vi "......SPEECH + GAIT + FACE  two command.vi"() -> ()   [LabVIEW 2018]
uses:
  <vilib>/Analysis/baseanly.llb/Mean (DBL).vi
  <vilib>/University of Leeds/Kinesthesia Toolkit for Microsoft Kinect/_Polymorphic Configure/Event-Skeleton and Video.vi
  <vilib>/Utility/file.llb/Read Delimited Spreadsheet (DBL).vi
  <vilib>/University of Leeds/Kinesthesia Toolkit for Microsoft Kinect/_Polymorphic Read/Read-Skeleton and Video.vi
  <vilib>/University of Leeds/Kinesthesia Toolkit for Microsoft Kinect/_Polymorphic Close/Close-Skeleton and Video.vi
  <vilib>/University of Leeds/Kinesthesia Toolkit for Microsoft Kinect/_Polymorphic Configure/Event-Video.vi
  <vilib>/University of Leeds/Kinesthesia Toolkit for Microsoft Kinect/_Polymorphic Read/Read-Video.vi
  <vilib>/University of Leeds/Kinesthesia Toolkit for Microsoft Kinect/_Polymorphic Close/Close-Video.vi
  <vilib>/Utility/file.llb/Write Delimited Spreadsheet (DBL).vi
  <vilib>/Analysis/NI_AALBase.lvlib
  <vilib>/vision/NI_Vision_Development_Module.lvlib
panel:
  in  "Eye Min Score":sgl=700.0
  in  "Nose Min Score":sgl=700.0
  in  "Lip Min Score":sgl=700.0
  out "Preview":T1(plugin-control)
  in  "Show Templates":bool
  out "Face Recognized?":bool
  out "Eye Template":T1(plugin-control)
  out "Nose Template":T1(plugin-control)
  out "Lips Template":T1(plugin-control)
  out "scan gait":refnum<vi>(3d-picture)
  out "Gait recognized?":bool
  out "real time data":dbl[](array[numeric])
  out "max mean":dbl[][](array[numeric])
  out "min mean":dbl[][](array[numeric])
  out "score":dbl
  out "mean calculated":dbl[](array[numeric])
  out "measure 3D":refnum<vi>(3d-picture)
  out "measure 2D":picture
  out "real time data":dbl[](array[numeric])
  in  "Error In":errorcluster
  out "Error Out":errorcluster
  in  "Exit":bool
  out "Speech Recognition":string
  # "Gait recognition"
  # "Set up user Gait info"
  # "Face recognition"
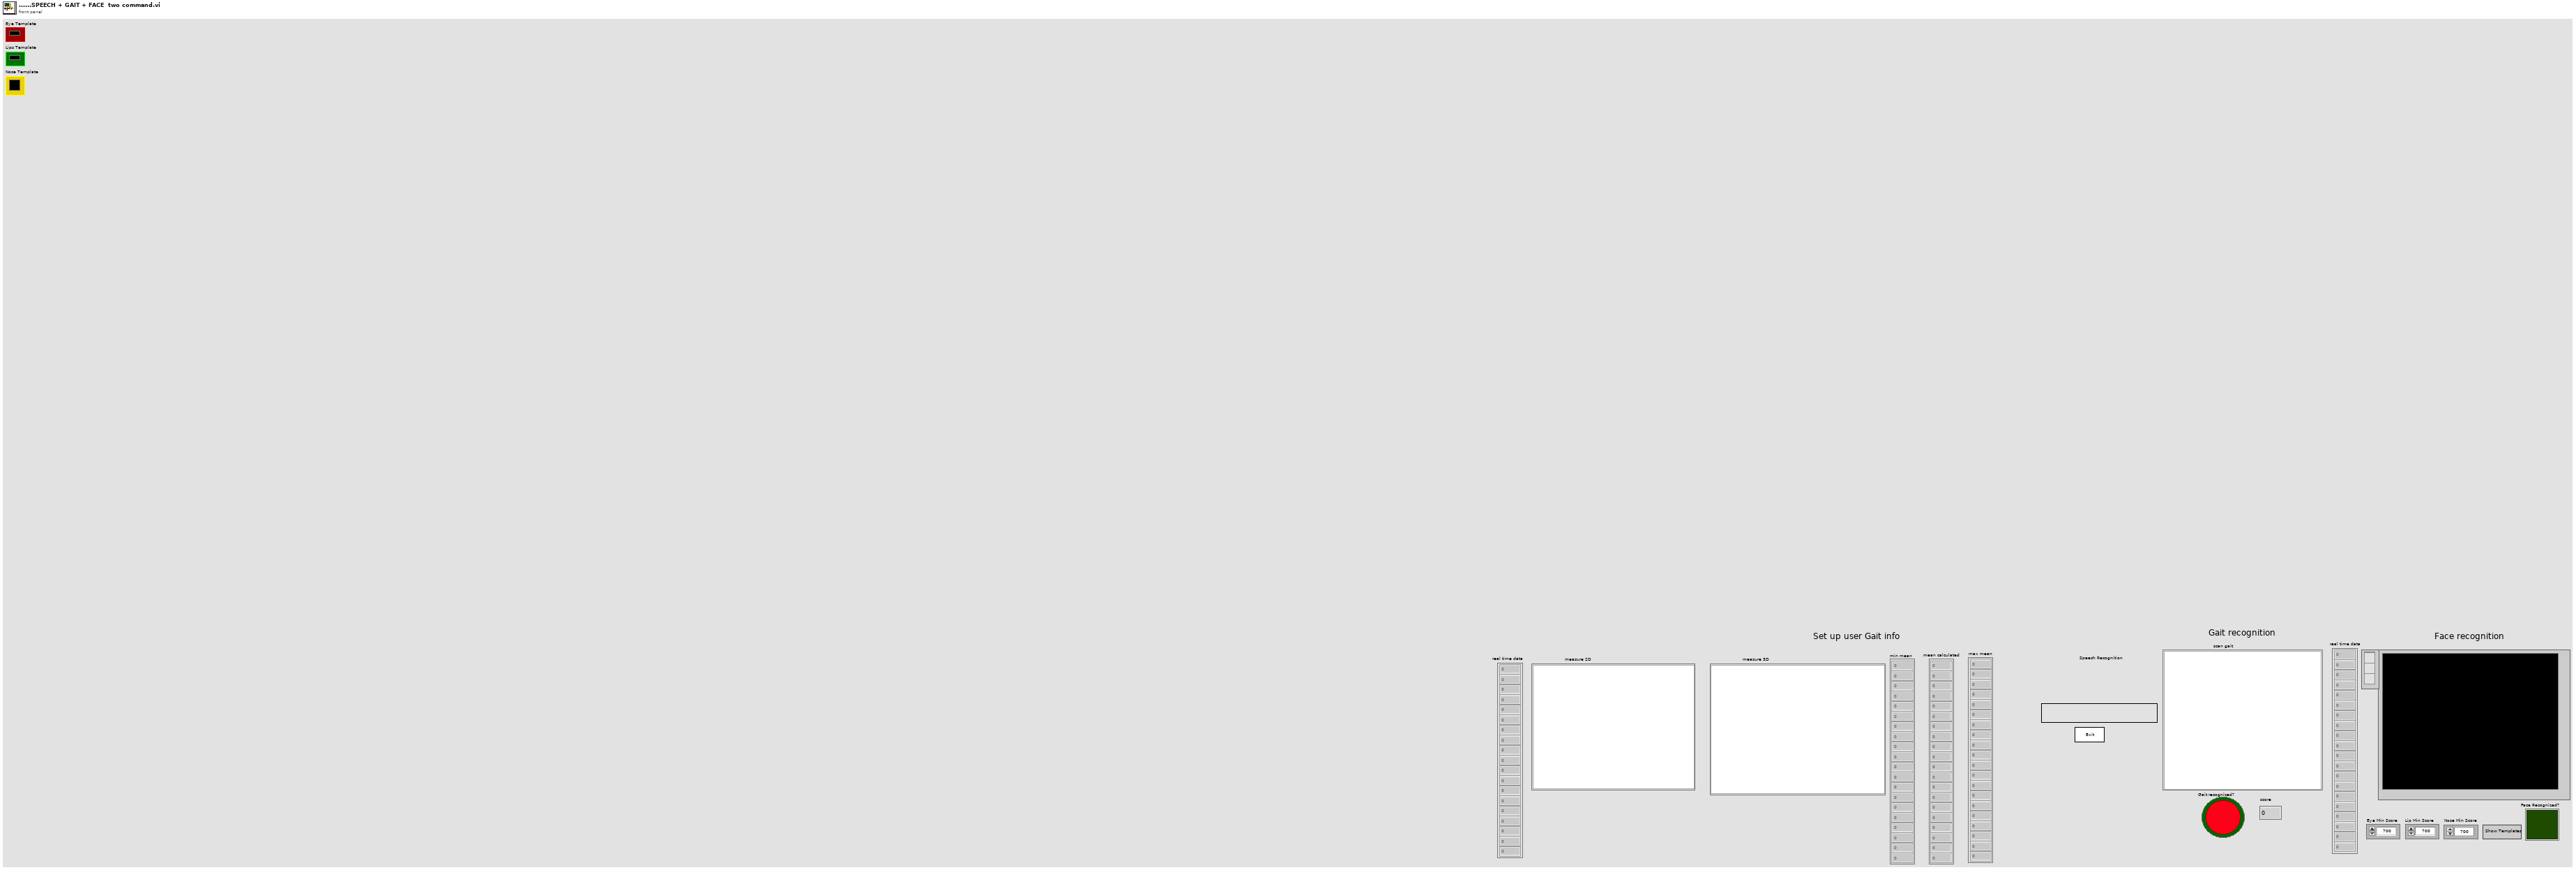
[diagram p1: front panel]
types:
  T1 = typedef "IMAQ Image.ctl" = refnum<image>
  T2 = enum16{"hip centre", "spine", "shoulder centre", "head", "shoulder left", "elbow left", "wrist left", "hand left", "shoulder right", "elbow right", "wrist right", "hand right", "hip left", "knee left", "ankle left", "foot left", "hip right", "knee right", "ankle right", "foot right"}
  T3 = cluster{cluster{"reference out":refnum<k24>, "KinectSensors":refnum<k24>}, "get_Item":refnum<k24>}
  T4 = cluster{"reference out":refnum<k24>, "KinectSensors":refnum<k24>, "SkeletonStream":refnum<k24>, "ColorStream":refnum<k24>, refnum<k24>[], "get_Item":refnum<k24>}
  T5 = cluster{"Scene":refnum<vi>, "Joints":refnum<vi>[], "Bones":refnum<vi>[]}
  T6 = cluster{"reference out":refnum<k24>, "KinectSensors":refnum<k24>, "ColorStream":refnum<k24>, "get_Item":refnum<k24>}
  T7 = typedef "Image Type" = u32
  T8 = cluster{"Position":cluster{"x":sgl, "y":sgl}, "Angle":sgl, "Scale":sgl, "Score":sgl, "Bounding Box":cluster{"x":sgl, "y":sgl}[]}[]
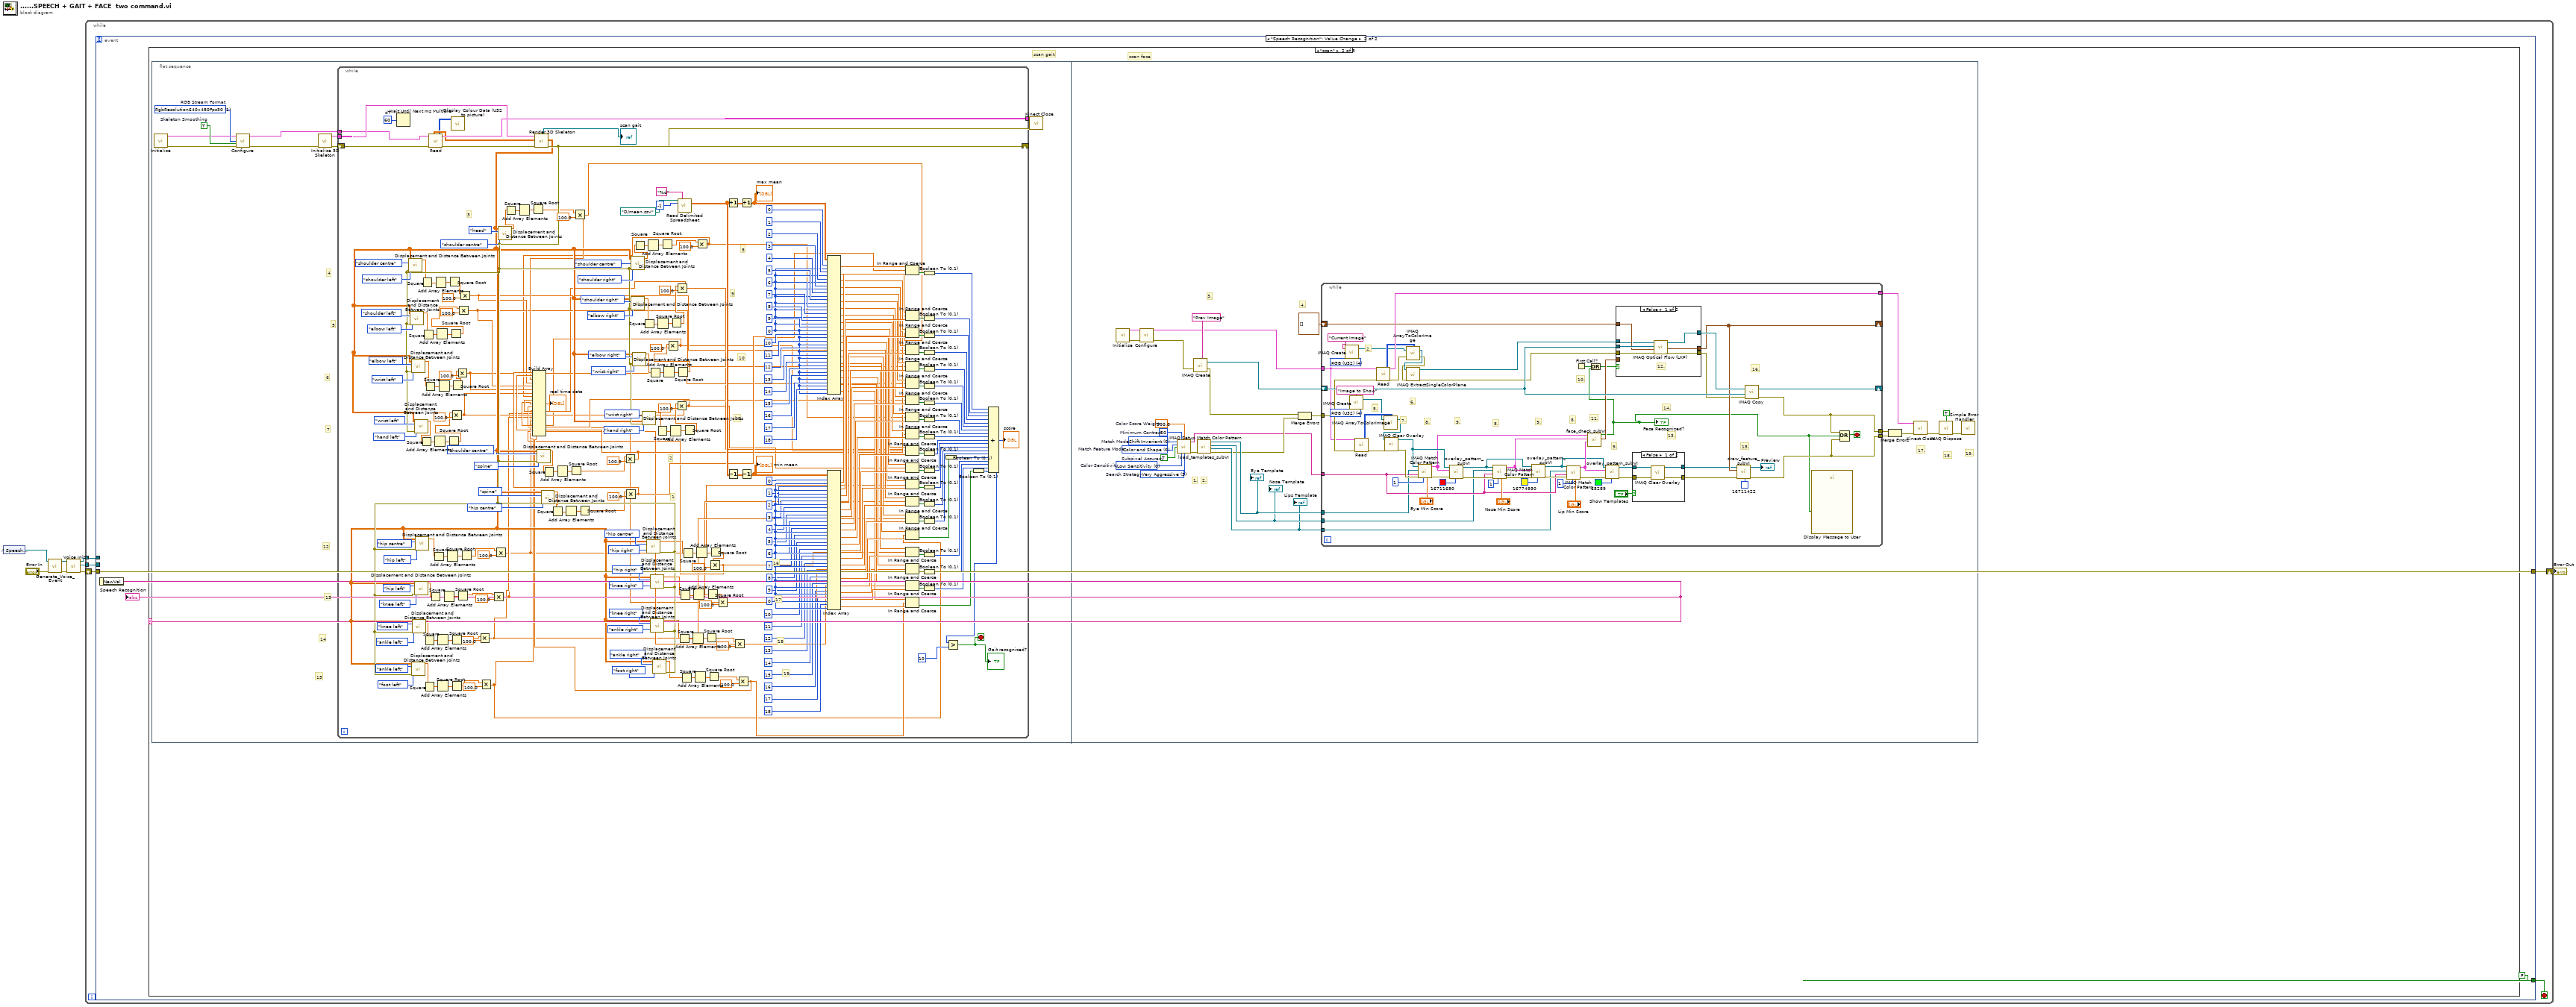
[diagram p0: block diagram]
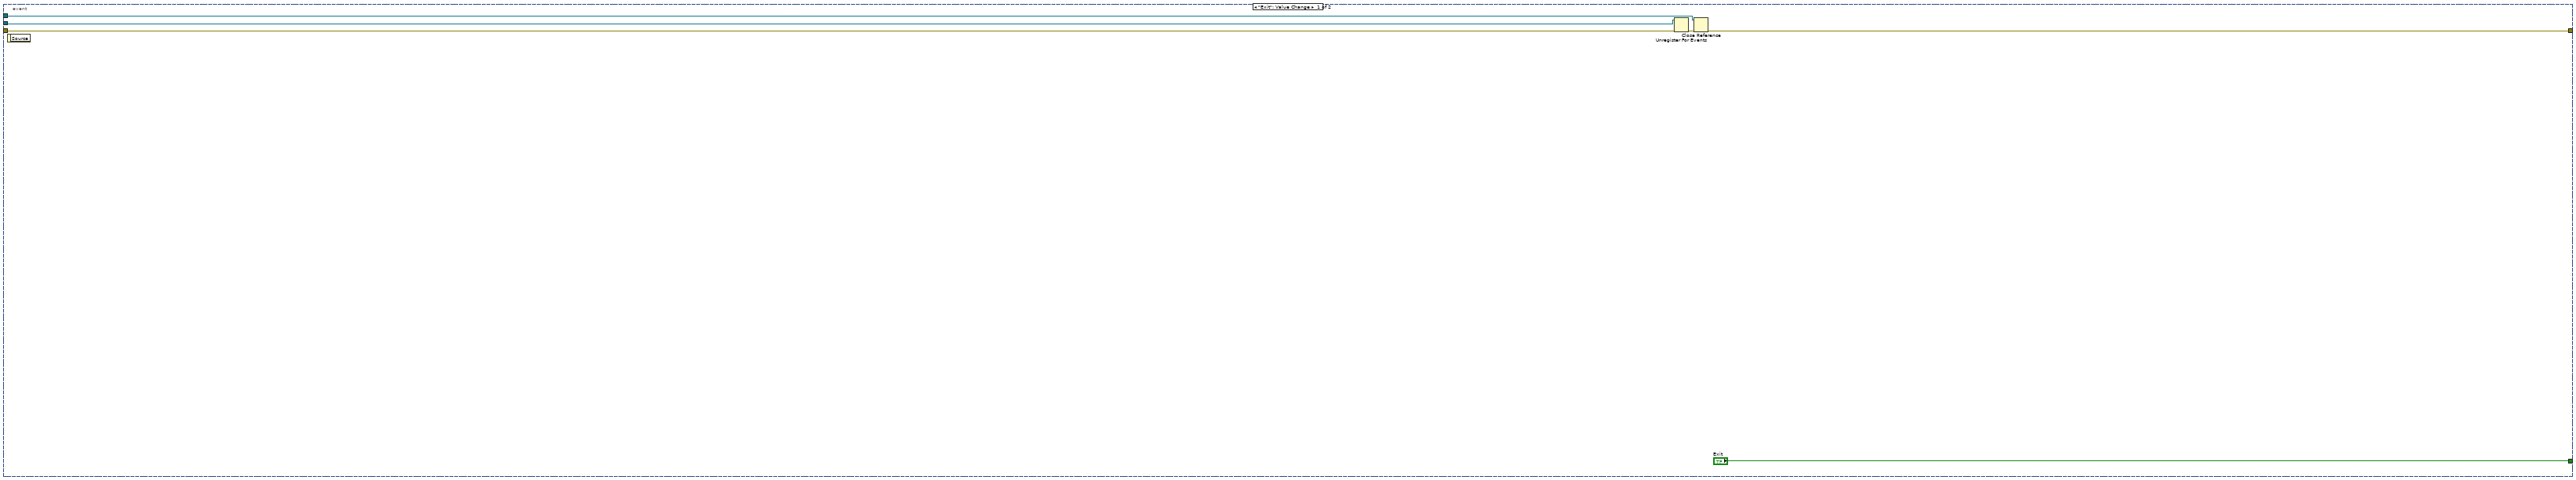
[diagram p2: hidden frame]
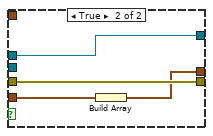
[diagram p5: hidden frame]
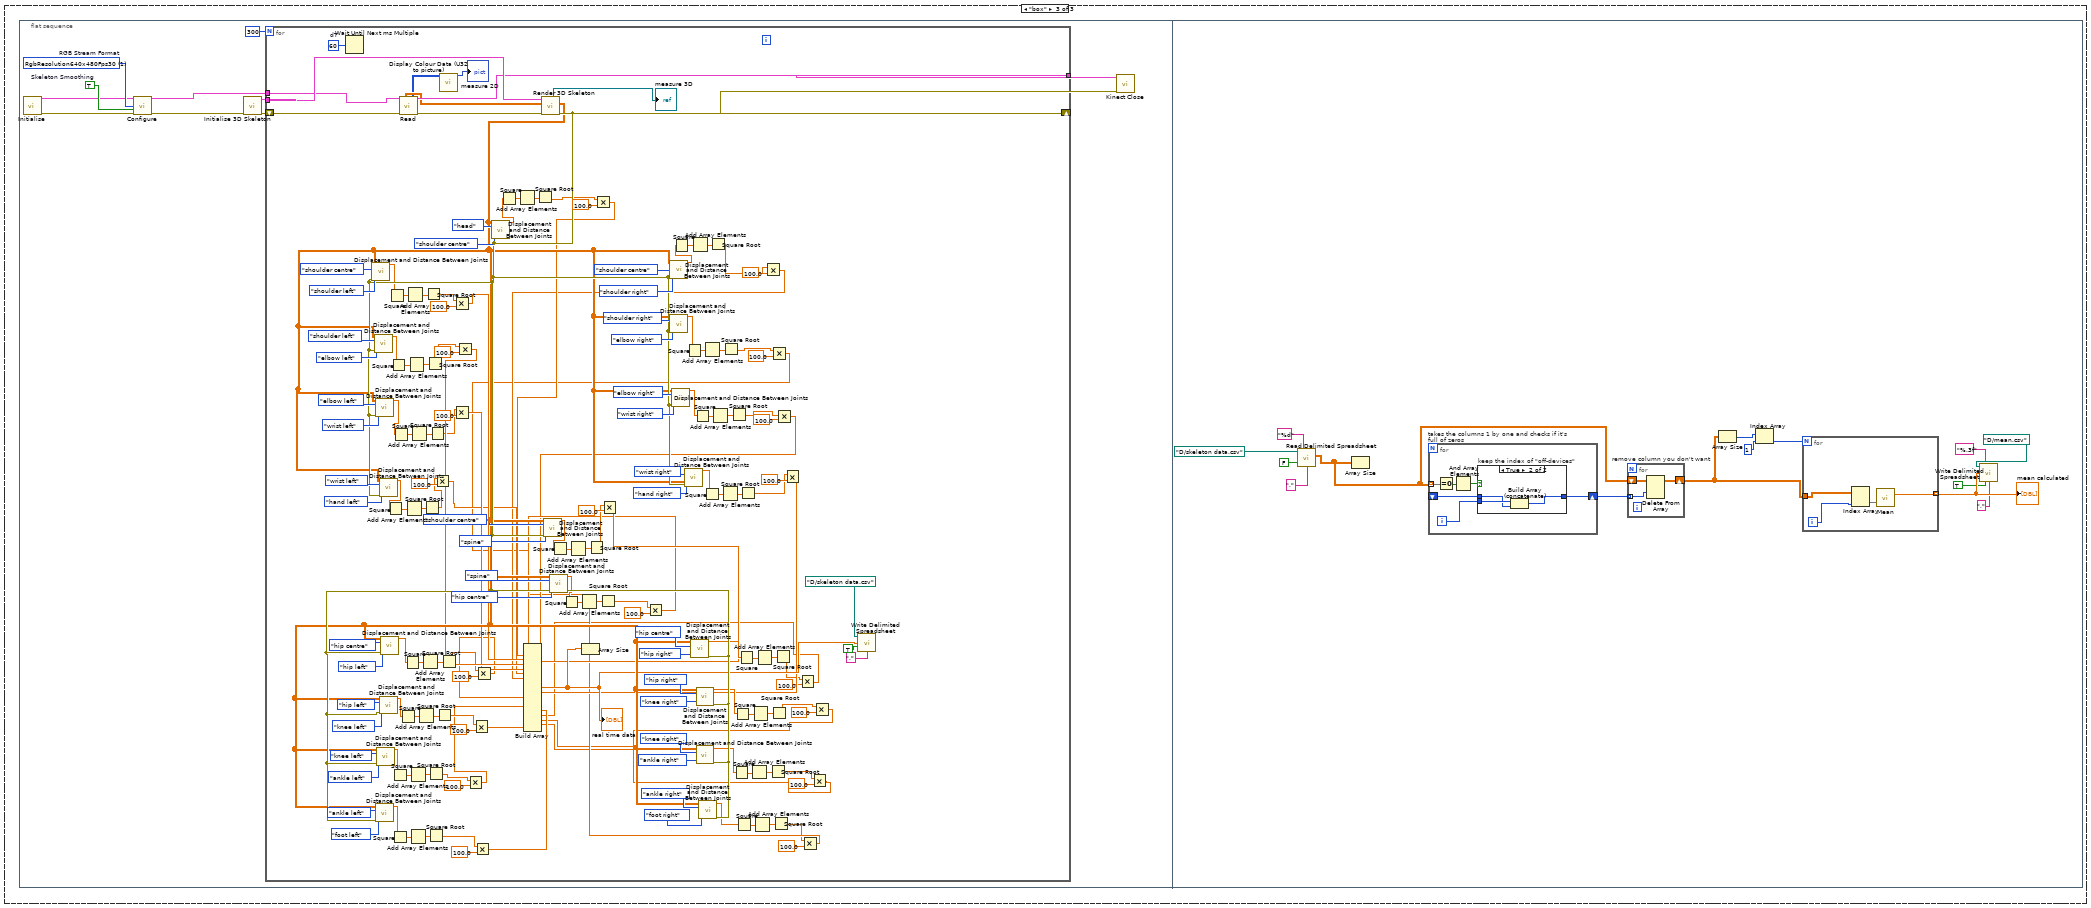
[diagram p6: hidden frame]
diagram:
  n1 = control-ref of="Speech Recognition"() -> (w7:refnum<vi>)
  n2 = call "Generate_Voice_Event.vi"("Error In"="Error In", "String in"=w7) -> ("Error Out"=w6:errorcluster, "String out"=w8:refnum<vi>)  [unwired: 8 in]
  n3 = call "Voice Init.vi"("Error In"=w6, "Text"=w8) -> ("Error Out"=w4:errorcluster, "Event Callback"=w1:refnum<k27>, "Reference"=w5:refnum<k24>)  [unwired: 7 in]
  n4 = while {
    tunnel: w5 -> [w12]
    shift-right: [w10] -> w3
    shift-left: w4 -> [w11]
    tunnel: w1 -> [w9]
    stop <- w13 stop-if-true
    n5 = event shown="[1] \"Speech Recognition\": Value Change" {
      selector: _ -> [_ _]
      dyn-events: _ -> [_ _]
      timeout: _ -> [_ _]
      tunnel: ["Exit" FALSE ("Exit")] -> w13
      tunnel: w12 -> [w18 _]
      tunnel: w11 -> [w16 w22]
      tunnel: [w15 w22] -> w10
      tunnel: w9 -> [w14 _]
      event "Exit": Value Change {
        n6 = event-data() -> ()  [unwired: 1 in, 1 out]
        n7 = Unregister For Events(event registration refnum=w14, error in=w16) -> (error out=w17:errorcluster)
        n8 = Close Reference(reference=w18, error in (no error)=w17) -> (error out=w15:errorcluster)
      }
      event "Speech Recognition": Value Change {
        n9 = event-data() -> ("NewVal"=w20:string)  [unwired: 1 in]
        "Speech Recognition" <- w20
        n10 = case shown="\"scan\"" w20 {
          frame Default {
          }
          frame "scan" {
            # "scan face"
            # "scan gait"
            n11 = flat-sequence {
              frame #0 {
                w28 = 1 items=["Undefined", "RgbResolution640x480Fps30", "RgbResolution1280x960Fps12", "YuvResolution640x480Fps15", "RawYuvResolution640x480Fps15"]  # RGB Stream Format
                w27 = TRUE  # Skeleton Smoothing
                # "15"
                # "14"
                # "13"
                # "12"
                # "7"
                # "6"
                # "5"
                # "4"
                n12 = call <vilib>:"Initialise.vi"() -> ("Kinect References out"=w23:T3, "error out"=w24:errorcluster)  [unwired: 14 in]
                n13 = call-poly <vilib>:"Configure.vi"("Kinect References in"=w23, "RGB Stream Format"=w28, "Skeleton Smoothing"=w27, "error in"=w24) -> ("Kinect References out"=w29:T4, "error out"=w30:errorcluster)  [unwired: 10 in]
                n14 = call <vilib>:"Initialise 3D Skeleton.vi"("error in (no error)"=w30) -> ("error out"=w31:errorcluster, "Scene & Skeleton Refs"=w32:T5)  [unwired: 9 in]
                n15 = while {
                  tunnel: [w317] -> w25
                  tunnel: w32 -> [w323]
                  tunnel: w29 -> [w318]
                  shift-right: [w276] -> w26
                  shift-left: w31 -> [w320]
                  stop <- w216 stop-if-true
                  w152 = 0 ("disabled index (col)")
                  w154 = 0 ("disabled index (col)")
                  w321 = u32 60  # dT
                  # "19"
                  # "18"
                  # "17"
                  # "16"
                  # "2"
                  # "1"
                  # "11"
                  # "10"
                  # "9"
                  # "8"
                  # "3"
                  n16 = Wait Until Next ms Multiple(millisecond multiple=w321) -> ()  [unwired: 1 out]
                  n17 = call-poly <vilib>:"Read.vi"("Kinect References in"=w318, "error in (no error)"=w320) -> ("Primary Skeleton Array"=w316:dbl[][], "Colour output array (U24, RGB)"=w315:u32[][], "Kinect References out"=w317:T4, "error out"=w319:errorcluster)  [unwired: 9 in, 1 out]
                  n18 = call <vilib>:"Display Colour Data (U32 to picture).vi"("Colour output array (U24, RGB)"=w315) -> ()  [unwired: 10 in, 1 out]
                  n19 = call <vilib>:"Render 3D Skeleton.vi"("error in (no error)"=w319, "Array of Joint Positions"=w316, "Scene & Skeleton Refs In"=w323) -> ("error out"=w276:errorcluster, "Array of Joint Positions Out"=w275:dbl[][], "Scene Out"=→"scan gait":refnum<vi>)  [unwired: 5 in, 1 out]
                  n20 = call <vilib>:"Displacement and Distance Between Joints.vi"("Array of Joint Positions"=w275, "Joint 1"=T2."shoulder centre", "Joint 2"=T2."shoulder left", "error in (no error)"=w276) -> ("X Y Z Displacement Between Joints 1 and 2"=w266:dbl[])  [unwired: 10 in, 1 out]
                  n21 = call <vilib>:"Displacement and Distance Between Joints.vi"("Array of Joint Positions"=w275, "Joint 1"=T2."shoulder left", "Joint 2"=T2."elbow left", "error in (no error)"=w276) -> ("X Y Z Displacement Between Joints 1 and 2"=w263:dbl[])  [unwired: 10 in, 1 out]
                  n22 = call <vilib>:"Displacement and Distance Between Joints.vi"("Array of Joint Positions"=w275, "Joint 1"=T2."elbow left", "Joint 2"=T2."wrist left", "error in (no error)"=w276) -> ("X Y Z Displacement Between Joints 1 and 2"=w257:dbl[])  [unwired: 10 in, 1 out]
                  n23 = call <vilib>:"Displacement and Distance Between Joints.vi"("Array of Joint Positions"=w275, "Joint 1"=T2."ankle left", "Joint 2"=T2."foot left", "error in (no error)"=w276) -> ("X Y Z Displacement Between Joints 1 and 2"=w230:dbl[])  [unwired: 10 in, 1 out]
                  n24 = call <vilib>:"Displacement and Distance Between Joints.vi"("Array of Joint Positions"=w275, "Joint 1"=T2."knee left", "Joint 2"=T2."ankle left", "error in (no error)"=w276) -> ("X Y Z Displacement Between Joints 1 and 2"=w231:dbl[])  [unwired: 10 in, 1 out]
                  n25 = call <vilib>:"Displacement and Distance Between Joints.vi"("Array of Joint Positions"=w275, "Joint 1"=T2."wrist left", "Joint 2"=T2."hand left", "error in (no error)"=w276) -> ("X Y Z Displacement Between Joints 1 and 2"=w247:dbl[])  [unwired: 10 in, 1 out]
                  n26 = call <vilib>:"Displacement and Distance Between Joints.vi"("Array of Joint Positions"=w275, "Joint 1"=T2."hip left", "Joint 2"=T2."knee left", "error in (no error)"=w276) -> ("X Y Z Displacement Between Joints 1 and 2"=w232:dbl[])  [unwired: 10 in, 1 out]
                  n27 = call <vilib>:"Displacement and Distance Between Joints.vi"("Array of Joint Positions"=w275, "Joint 1"=T2."hip centre", "Joint 2"=T2."hip left", "error in (no error)"=w276) -> ("X Y Z Displacement Between Joints 1 and 2"=w239:dbl[])  [unwired: 10 in, 1 out]
                  n28 = Square(x=w247) -> (x^2=w251:dbl[])
                  n29 = Square(x=w266) -> (x^2=w268:dbl[])
                  n30 = Square(x=w263) -> (x^2=w265:dbl[])
                  n31 = Square(x=w231) -> (x^2=w236:dbl[])
                  n32 = Square(x=w230) -> (x^2=w234:dbl[])
                  n33 = Square(x=w257) -> (x^2=w259:dbl[])
                  n34 = Square(x=w232) -> (x^2=w238:dbl[])
                  n35 = Square(x=w239) -> (x^2=w241:dbl[])
                  n36 = Add Array Elements(numeric array=w251) -> (sum=w250:dbl)
                  n37 = Add Array Elements(numeric array=w268) -> (sum=w267:dbl)
                  n38 = Add Array Elements(numeric array=w265) -> (sum=w264:dbl)
                  n39 = Add Array Elements(numeric array=w236) -> (sum=w235:dbl)
                  n40 = Add Array Elements(numeric array=w234) -> (sum=w233:dbl)
                  n41 = Add Array Elements(numeric array=w259) -> (sum=w258:dbl)
                  n42 = Add Array Elements(numeric array=w238) -> (sum=w237:dbl)
                  n43 = Add Array Elements(numeric array=w241) -> (sum=w240:dbl)
                  n44 = Square Root(x=w250) -> (sqrt(x)=w206:dbl)
                  n45 = Square Root(x=w267) -> (sqrt(x)=w214:dbl)
                  n46 = Square Root(x=w264) -> (sqrt(x)=w210:dbl)
                  n47 = Multiply(x=w206, y=100.0) -> (x*y=w46:dbl)
                  n48 = Square Root(x=w235) -> (sqrt(x)=w188:dbl)
                  n49 = Square Root(x=w233) -> (sqrt(x)=w186:dbl)
                  n50 = Square Root(x=w258) -> (sqrt(x)=w208:dbl)
                  n51 = Multiply(x=w208, y=100.0) -> (x*y=w47:dbl)
                  n52 = Square Root(x=w237) -> (sqrt(x)=w190:dbl)
                  n53 = Multiply(x=w210, y=100.0) -> (x*y=w48:dbl)
                  n54 = Multiply(x=w214, y=100.0) -> (x*y=w49:dbl)
                  n55 = Square Root(x=w240) -> (sqrt(x)=w192:dbl)
                  n56 = Multiply(x=w188, y=100.0) -> (x*y=w36:dbl)
                  n57 = Multiply(x=w186, y=100.0) -> (x*y=w37:dbl)
                  n58 = Multiply(x=w190, y=100.0) -> (x*y=w35:dbl)
                  n59 = Multiply(x=w192, y=100.0) -> (x*y=w34:dbl)
                  n60 = call <vilib>:"Displacement and Distance Between Joints.vi"("Array of Joint Positions"=w275, "Joint 1"=T2."head", "Joint 2"=T2."shoulder centre", "error in (no error)"=w276) -> ("X Y Z Displacement Between Joints 1 and 2"=w272:dbl[])  [unwired: 10 in, 1 out]
                  n61 = Square(x=w272) -> (x^2=w274:dbl[])
                  n62 = Add Array Elements(numeric array=w274) -> (sum=w273:dbl)
                  n63 = Square Root(x=w273) -> (sqrt(x)=w212:dbl)
                  n64 = call <vilib>:"Displacement and Distance Between Joints.vi"("Array of Joint Positions"=w275, "Joint 1"=T2."shoulder centre", "Joint 2"=T2."spine", "error in (no error)"=w276) -> ("X Y Z Displacement Between Joints 1 and 2"=w245:dbl[])  [unwired: 10 in, 1 out]
                  n65 = call <vilib>:"Displacement and Distance Between Joints.vi"("Array of Joint Positions"=w275, "Joint 1"=T2."spine", "Joint 2"=T2."hip centre", "error in (no error)"=w276) -> ("X Y Z Displacement Between Joints 1 and 2"=w242:dbl[])  [unwired: 10 in, 1 out]
                  n66 = Square(x=w245) -> (x^2=w253:dbl[])
                  n67 = Square(x=w242) -> (x^2=w244:dbl[])
                  n68 = Add Array Elements(numeric array=w253) -> (sum=w252:dbl)
                  n69 = Add Array Elements(numeric array=w244) -> (sum=w243:dbl)
                  n70 = Square Root(x=w252) -> (sqrt(x)=w204:dbl)
                  n71 = Multiply(x=w212, y=100.0) -> (x*y=w50:dbl)
                  n72 = Square Root(x=w243) -> (sqrt(x)=w194:dbl)
                  n73 = Multiply(x=w204, y=100.0) -> (x*y=w51:dbl)
                  n74 = Multiply(x=w194, y=100.0) -> (x*y=w52:dbl)
                  n75 = call <vilib>:"Displacement and Distance Between Joints.vi"("Array of Joint Positions"=w275, "Joint 1"=T2."shoulder centre", "Joint 2"=T2."shoulder right", "error in (no error)"=w276) -> ("X Y Z Displacement Between Joints 1 and 2"=w269:dbl[])  [unwired: 10 in, 1 out]
                  n76 = call <vilib>:"Displacement and Distance Between Joints.vi"("Array of Joint Positions"=w275, "Joint 1"=T2."shoulder right", "Joint 2"=T2."elbow right", "error in (no error)"=w276) -> ("X Y Z Displacement Between Joints 1 and 2"=w260:dbl[])  [unwired: 10 in, 1 out]
                  n77 = call <vilib>:"Displacement and Distance Between Joints.vi"("Array of Joint Positions"=w275, "Joint 1"=T2."elbow right", "Joint 2"=T2."wrist right", "error in (no error)"=w276) -> ("X Y Z Displacement Between Joints 1 and 2"=w254:dbl[])  [unwired: 10 in, 1 out]
                  n78 = Square(x=w269) -> (x^2=w271:dbl[])
                  n79 = call <vilib>:"Displacement and Distance Between Joints.vi"("Array of Joint Positions"=w275, "Joint 1"=T2."wrist right", "Joint 2"=T2."hand right", "error in (no error)"=w276) -> ("X Y Z Displacement Between Joints 1 and 2"=w246:dbl[])  [unwired: 10 in, 1 out]
                  n80 = Square(x=w260) -> (x^2=w262:dbl[])
                  n81 = Add Array Elements(numeric array=w271) -> (sum=w270:dbl)
                  n82 = call <vilib>:"Displacement and Distance Between Joints.vi"("Array of Joint Positions"=w275, "Joint 1"=T2."hip centre", "Joint 2"=T2."hip right", "error in (no error)"=w276) -> ("X Y Z Displacement Between Joints 1 and 2"=w227:dbl[])  [unwired: 10 in, 1 out]
                  n83 = Square(x=w254) -> (x^2=w256:dbl[])
                  n84 = call <vilib>:"Displacement and Distance Between Joints.vi"("Array of Joint Positions"=w275, "Joint 1"=T2."hip right", "Joint 2"=T2."knee right", "error in (no error)"=w276) -> ("X Y Z Displacement Between Joints 1 and 2"=w220:dbl[])  [unwired: 10 in, 1 out]
                  n85 = call <vilib>:"Displacement and Distance Between Joints.vi"("Array of Joint Positions"=w275, "Joint 1"=T2."knee right", "Joint 2"=T2."ankle right", "error in (no error)"=w276) -> ("X Y Z Displacement Between Joints 1 and 2"=w219:dbl[])  [unwired: 10 in, 1 out]
                  n86 = call <vilib>:"Displacement and Distance Between Joints.vi"("Array of Joint Positions"=w275, "Joint 1"=T2."ankle right", "Joint 2"=T2."foot right", "error in (no error)"=w276) -> ("X Y Z Displacement Between Joints 1 and 2"=w218:dbl[])  [unwired: 10 in, 1 out]
                  n87 = Square(x=w246) -> (x^2=w249:dbl[])
                  n88 = Add Array Elements(numeric array=w262) -> (sum=w261:dbl)
                  n89 = Square Root(x=w270) -> (sqrt(x)=w202:dbl)
                  n90 = Add Array Elements(numeric array=w256) -> (sum=w255:dbl)
                  n91 = Add Array Elements(numeric array=w249) -> (sum=w248:dbl)
                  n92 = Square Root(x=w261) -> (sqrt(x)=w200:dbl)
                  n93 = Multiply(x=w200, y=100.0) -> (x*y=w44:dbl)
                  n94 = Square Root(x=w255) -> (sqrt(x)=w198:dbl)
                  n95 = Multiply(x=w198, y=100.0) -> (x*y=w43:dbl)
                  n96 = call-poly <vilib>:"Read Delimited Spreadsheet.vi"("file path (dialog if empty)"=path "D:/mean.csv" ("file path"), "format (%.3f)"="%d", "number of rows (all:-1)"=-1) -> ("all rows"=w130:dbl[][])  [unwired: 7 in, 5 out]
                  n97 = Square(x=w219) -> (x^2=w224:dbl[])
                  n98 = Square(x=w220) -> (x^2=w226:dbl[])
                  n99 = Square(x=w218) -> (x^2=w221:dbl[])
                  n100 = Square(x=w227) -> (x^2=w229:dbl[])
                  n101 = Square Root(x=w248) -> (sqrt(x)=w196:dbl)
                  n102 = Multiply(x=w196, y=100.0) -> (x*y=w42:dbl)
                  n103 = Add Array Elements(numeric array=w224) -> (sum=w223:dbl)
                  n104 = Add Array Elements(numeric array=w226) -> (sum=w225:dbl)
                  n105 = Add Array Elements(numeric array=w221) -> (sum=w222:dbl)
                  n106 = Add Array Elements(numeric array=w229) -> (sum=w228:dbl)
                  n107 = Multiply(x=w202, y=100.0) -> (x*y=w45:dbl)
                  n108 = Square Root(x=w223) -> (sqrt(x)=w182:dbl)
                  n109 = Square Root(x=w225) -> (sqrt(x)=w180:dbl)
                  n110 = Square Root(x=w222) -> (sqrt(x)=w184:dbl)
                  n111 = Square Root(x=w228) -> (sqrt(x)=w178:dbl)
                  n112 = Multiply(x=w178, y=100.0) -> (x*y=w38:dbl)
                  n113 = Multiply(x=w180, y=100.0) -> (x*y=w39:dbl)
                  n114 = Increment(x=w130) -> (x+1=w129:dbl[][])
                  n115 = Decrement(x=w130) -> (x-1=w131:dbl[][])
                  n116 = Multiply(x=w182, y=100.0) -> (x*y=w40:dbl)
                  n117 = Multiply(x=w184, y=100.0) -> (x*y=w41:dbl)
                  n118 = Build Array(w52, w51, w50, w49, w48, w47, w46, w45, w44, w43, w42, w34, w35, w36, w37, w38, w39, w40, w41) -> (→"real time data":dbl[])
                  n119 = Increment(x=w129) -> (x+1=w153:dbl[][])
                  "max mean" <- w153
                  n120 = Decrement(x=w131) -> (x-1=w132:dbl[][])
                  "min mean" <- w132
                  n121 = Index Array(array=w153, index (row) #1=0 ("disabled index (row)"), index (col) #1=w154, index (row) #2=1 ("disabled index (row)"), index (col) #2=w154, index (row) #3=2 ("disabled index (row)"), index (col) #3=w154, index (row) #4=3 ("disabled index (row)"), index (col) #4=w154, index (row) #5=4 ("disabled index (row)"), index (col) #5=w154, index (row) #6=5 ("disabled index (row)"), index (col) #6=w154, index (row) #7=6 ("disabled index (row)"), index (col) #7=w154, index (row) #8=7 ("disabled index (row)"), index (col) #8=w154, index (row) #9=8 ("disabled index (row)"), index (col) #9=w154, index (row) #10=9 ("disabled index (row)"), index (col) #10=w154, index (row) #11=10 ("disabled index (row)"), index (col) #11=w154, index (row) #12=11 ("disabled index (row)"), index (col) #12=w154, index (row) #13=12 ("disabled index (row)"), index (col) #13=w154, index (row) #14=13 ("disabled index (row)"), index (col) #14=w154, index (row) #15=14 ("disabled index (row)"), index (col) #15=w154, index (row) #16=15 ("disabled index (row)"), index (col) #16=w154, index (row) #17=16 ("disabled index (row)"), index (col) #17=w154, index (row) #18=17 ("disabled index (row)"), index (col) #18=w154, index (row) #19=18 ("disabled index (row)"), index (col) #19=w154) -> (element #1=w92:dbl, element #2=w72:dbl, element #3=w71:dbl, element #4=w70:dbl, element #5=w69:dbl, element #6=w68:dbl, element #7=w67:dbl, element #8=w66:dbl, element #9=w65:dbl, element #10=w64:dbl, element #11=w55:dbl, element #12=w56:dbl, element #13=w57:dbl, element #14=w58:dbl, element #15=w59:dbl, element #16=w60:dbl, element #17=w61:dbl, element #18=w62:dbl, element #19=w63:dbl)
                  n122 = Index Array(array=w132, index (row) #1=0 ("disabled index (row)"), index (col) #1=w152, index (row) #2=1 ("disabled index (row)"), index (col) #2=w152, index (row) #3=2 ("disabled index (row)"), index (col) #3=w152, index (row) #4=3 ("disabled index (row)"), index (col) #4=w152, index (row) #5=4 ("disabled index (row)"), index (col) #5=w152, index (row) #6=5 ("disabled index (row)"), index (col) #6=w152, index (row) #7=6 ("disabled index (row)"), index (col) #7=w152, index (row) #8=7 ("disabled index (row)"), index (col) #8=w152, index (row) #9=8 ("disabled index (row)"), index (col) #9=w152, index (row) #10=9 ("disabled index (row)"), index (col) #10=w152, index (row) #11=10 ("disabled index (row)"), index (col) #11=w152, index (row) #12=11 ("disabled index (row)"), index (col) #12=w152, index (row) #13=12 ("disabled index (row)"), index (col) #13=w152, index (row) #14=13 ("disabled index (row)"), index (col) #14=w152, index (row) #15=14 ("disabled index (row)"), index (col) #15=w152, index (row) #16=15 ("disabled index (row)"), index (col) #16=w152, index (row) #17=16 ("disabled index (row)"), index (col) #17=w152, index (row) #18=17 ("disabled index (row)"), index (col) #18=w152, index (row) #19=18 ("disabled index (row)"), index (col) #19=w152) -> (element #1=w91:dbl, element #2=w90:dbl, element #3=w89:dbl, element #4=w88:dbl, element #5=w87:dbl, element #6=w86:dbl, element #7=w85:dbl, element #8=w84:dbl, element #9=w83:dbl, element #10=w82:dbl, element #11=w81:dbl, element #12=w80:dbl, element #13=w79:dbl, element #14=w78:dbl, element #15=w77:dbl, element #16=w76:dbl, element #17=w75:dbl, element #18=w74:dbl, element #19=w73:dbl)
                  n123 = In Range and Coerce(upper limit=w92, x=w52, lower limit=w91) -> (In Range?=w128:bool)  [unwired: 1 out]
                  n124 = In Range and Coerce(upper limit=w72, x=w51, lower limit=w90) -> (In Range?=w127:bool)  [unwired: 1 out]
                  n125 = In Range and Coerce(upper limit=w71, x=w50, lower limit=w89) -> (In Range?=w126:bool)  [unwired: 1 out]
                  n126 = In Range and Coerce(upper limit=w70, x=w49, lower limit=w88) -> (In Range?=w125:bool)  [unwired: 1 out]
                  n127 = In Range and Coerce(upper limit=w69, x=w48, lower limit=w87) -> (In Range?=w124:bool)  [unwired: 1 out]
                  n128 = In Range and Coerce(upper limit=w68, x=w47, lower limit=w86) -> (In Range?=w123:bool)  [unwired: 1 out]
                  n129 = In Range and Coerce(upper limit=w67, x=w46, lower limit=w85) -> (In Range?=w122:bool)  [unwired: 1 out]
                  n130 = In Range and Coerce(upper limit=w66, x=w45, lower limit=w84) -> (In Range?=w121:bool)  [unwired: 1 out]
                  n131 = In Range and Coerce(upper limit=w65, x=w44, lower limit=w83) -> (In Range?=w120:bool)  [unwired: 1 out]
                  n132 = In Range and Coerce(upper limit=w64, x=w43, lower limit=w82) -> (In Range?=w119:bool)  [unwired: 1 out]
                  n133 = In Range and Coerce(upper limit=w55, x=w42, lower limit=w81) -> (In Range?=w118:bool)  [unwired: 1 out]
                  n134 = In Range and Coerce(upper limit=w56, x=w34, lower limit=w80) -> (In Range?=w117:bool)  [unwired: 1 out]
                  n135 = In Range and Coerce(upper limit=w57, x=w35, lower limit=w79) -> (In Range?=w116:bool)  [unwired: 1 out]
                  n136 = In Range and Coerce(upper limit=w58, x=w36, lower limit=w78) -> (In Range?=w115:bool)  [unwired: 1 out]
                  n137 = In Range and Coerce(upper limit=w59, x=w37, lower limit=w77) -> (In Range?=w53:bool)  [unwired: 1 out]
                  n138 = In Range and Coerce(upper limit=w60, x=w38, lower limit=w76) -> (In Range?=w114:bool)  [unwired: 1 out]
                  n139 = In Range and Coerce(upper limit=w61, x=w39, lower limit=w75) -> (In Range?=w113:bool)  [unwired: 1 out]
                  n140 = In Range and Coerce(upper limit=w62, x=w40, lower limit=w74) -> (In Range?=w112:bool)  [unwired: 1 out]
                  n141 = In Range and Coerce(upper limit=w63, x=w41, lower limit=w73) -> (In Range?=w54:bool)  [unwired: 1 out]
                  n142 = Boolean To (0,1)(Boolean=w128) -> (0, 1=w111:i16)
                  n143 = Boolean To (0,1)(Boolean=w127) -> (0, 1=w110:i16)
                  n144 = Boolean To (0,1)(Boolean=w126) -> (0, 1=w109:i16)
                  n145 = Boolean To (0,1)(Boolean=w125) -> (0, 1=w108:i16)
                  n146 = Boolean To (0,1)(Boolean=w124) -> (0, 1=w107:i16)
                  n147 = Boolean To (0,1)(Boolean=w123) -> (0, 1=w106:i16)
                  n148 = Boolean To (0,1)(Boolean=w122) -> (0, 1=w105:i16)
                  n149 = Boolean To (0,1)(Boolean=w121) -> (0, 1=w104:i16)
                  n150 = Boolean To (0,1)(Boolean=w120) -> (0, 1=w103:i16)
                  n151 = Boolean To (0,1)(Boolean=w119) -> (0, 1=w102:i16)
                  n152 = Boolean To (0,1)(Boolean=w118) -> (0, 1=w101:i16)
                  n153 = Boolean To (0,1)(Boolean=w117) -> (0, 1=w100:i16)
                  n154 = Boolean To (0,1)(Boolean=w116) -> (0, 1=w99:i16)
                  n155 = Boolean To (0,1)(Boolean=w115) -> (0, 1=w98:i16)
                  n156 = Boolean To (0,1)(Boolean=w114) -> (0, 1=w96:i16)
                  n157 = Boolean To (0,1)(Boolean=w113) -> (0, 1=w95:i16)
                  n158 = Boolean To (0,1)(Boolean=w112) -> (0, 1=w94:i16)
                  n159 = Boolean To (0,1)(Boolean=w53) -> (0, 1=w97:i16)
                  n160 = Boolean To (0,1)(Boolean=w54) -> (0, 1=w93:i16)
                  n161 = Compound Arithmetic op=ADD(w111, w110, w109, w108, w107, w106, w105, w104, w103, w102, w101, w100, w99, w98, w97, w96, w95, w94, w93) -> (w33:i16)
                  "score" <- w33
                  n162 = Greater?(x=w33, y=i16 10) -> (0:w216:bool)
                  "Gait recognized?" <- w216
                }
                n163 = call-poly <vilib>:"Kinect Close.vi"("Kinect References in"=w25, "error in"=w26) -> ()  [unwired: 13 in, 1 out]
              }
              frame #1 {
                w339 = TRUE  # Subpixel Accuracy
                w345 = u32 0 items=["Color and Shape", "Color", "Shape"]  # Match Feature Mode
                w344 = u32 3 items=["Conservative", "Balance", "Aggressive", "Very Aggressive"]  # Search Strategy
                w343 = 20  # Minimum Contrast
                w342 = sgl 300.0  # Color Score Weight
                w341 = u32 0 items=["Low Sensitivity", "Medium Sensitivity", "High Sensitivity"]  # Color Sensitivity
                w340 = u32 0 items=["Shift Invariant", "Rotation Invariant"]  # Match Mode
                # "19."
                # "17."
                # "4."
                # "3."
                # "3."
                # "3."
                # "2."
                # "1."
                # "18."
                n164 = call <vilib>:"Initialise.vi"() -> ("Kinect References out"=w350:T3, "error out"=w349:errorcluster)  [unwired: 14 in]
                n165 = call-poly <vilib>:"Configure.vi"("Kinect References in"=w350, "error in"=w349) -> ("Kinect References out"=w346:T6, "error out"=w325:errorcluster)  [unwired: 12 in]
                n166 = call "IMAQ Setup Match Color Pattern"("Match Mode"=w340, "Minimum Contrast"=w343, "Color Score Weight"=w342, "Match Feature Mode"=w345, "Subpixel Accuracy"=w339, "Color Sensitivity"=w341, "Search Strategy"=w344) -> ("Match Color Pattern Setup Data"=w329:string, "error out"=w338:errorcluster)  [unwired: 7 in]
                n167 = call "IMAQ Create"("Image Name"="Prev Image", "error in (no error)"=w325) -> ("New Image"=w347:T1, "error out"=w324:errorcluster)  [unwired: 2 in, 1 out]
                n168 = call "load_templates_subVI.vi"("error in (no error)"=w338) -> ("error out"=w331:errorcluster, "Lips Template"=w335:T1, "Nose Template"=w336:T1, "Eye Template"=w337:T1)  [unwired: 7 in]
                "Eye Template" <- w337
                "Nose Template" <- w336
                "Lips Template" <- w335
                n169 = Merge Errors(w324, w331) -> (w330:errorcluster)
                n170 = while {
                  shift-right: [w414] -> _
                  shift-left: w347 -> [w415]
                  shift-right: [w380] -> _
                  shift-left: cluster{"X":sgl, "Y":sgl}[] [] ("Feature Points Out") -> [w413]
                  tunnel: w346 -> [w371]
                  tunnel: [w412] -> w351
                  tunnel: w329 -> [w387]
                  tunnel: w337 -> [w386]
                  tunnel: w336 -> [w385]
                  tunnel: w335 -> [w384]
                  tunnel: w330 -> [w373]
                  tunnel: [w369] -> w328
                  tunnel: [w368] -> w327
                  stop <- w370 stop-if-true
                  w355 = T7 4 items=["Grayscale (U8)", "Grayscale (I16)", "Grayscale (SGL)", "Complex (CSG)", "RGB (U32)", "HSL (U32)", "RGB (U64)", "Grayscale (U16)"] ("Image Type")
                  w357 = T7 4 items=["Grayscale (U8)", "Grayscale (I16)", "Grayscale (SGL)", "Complex (CSG)", "RGB (U32)", "HSL (U32)", "RGB (U64)", "Grayscale (U16)"] ("Image Type")
                  # "4."
                  # "2."
                  # "10."
                  # "16."
                  # "15."
                  # "14."
                  # "13."
                  # "11."
                  # "9."
                  # "8."
                  # "9."
                  # "8."
                  # "9."
                  # "8."
                  # "7."
                  # "6."
                  # "5."
                  # "5."
                  n171 = call "IMAQ Create"("Image Name"="Current Image", "Image Type"=w355) -> ("New Image"=w359:T1)  [unwired: 2 in, 2 out]
                  n172 = call "IMAQ Create"("Image Name"="Image to Show", "Image Type"=w357) -> ("New Image"=w354:T1)  [unwired: 2 in, 2 out]
                  n173 = call-poly <vilib>:"Read.vi"("Kinect References in"=w371, "error in (no error)"=w373) -> ("Colour output array (U24, RGB)"=w363:u32[][], "error out"=w382:errorcluster)  [unwired: 10 in, 2 out]
                  n174 = call-poly <vilib>:"Read.vi"("Kinect References in"=w371, "error in (no error)"=w373) -> ("Colour output array (U24, RGB)"=w365:u32[][], "Kinect References out"=w412:T6, "error out"=w361:errorcluster)  [unwired: 10 in, 1 out]
                  n175 = call "IMAQ ArrayToColorImage"("Image Pixels (U32)"=w363, "Image"=w354) -> ("Image Out"=w362:T1)  [unwired: 3 in, 1 out]
                  n176 = call "IMAQ Clear Overlay"("error in (no error)"=w382, "Image"=w362) -> ("error out"=w408:errorcluster, "Image Out"=w394:T1)  [unwired: 8 in]
                  n177 = call "IMAQ ArrayToColorImage"("Image Pixels (U32)"=w365, "Image"=w359, "error in (no error)"=w361) -> ("Image Out"=w364:T1, "error out"=w360:errorcluster)  [unwired: 2 in]
                  n178 = call "IMAQ ExtractSingleColorPlane"("error in (no error)"=w360, "Image Src"=w364) -> ("error out"=w411:errorcluster, "Image Dst Out"=w410:T1)  [unwired: 8 in]
                  n179 = call "IMAQ Match Color Pattern"("Minimum Match Score"="Eye Min Score", "Number of Matches Requested"=1, "error in (no error)"=w408, "Match Color Pattern Setup Data"=w387, "Template Image"=w386, "Image"=w394) -> ("error out"=w407:errorcluster, "Matches"=w391:T8)  [unwired: 3 in, 1 out]
                  n180 = call "overlay_pattern_subVI.vi"("Color"=u32 16711680, "error in"=w407, "Matches"=w391, "Image"=w394) -> ("error out"=w404:errorcluster, "Image Out"=w401:T1)  [unwired: 6 in]
                  n181 = call "IMAQ Match Color Pattern"("Minimum Match Score"="Nose Min Score", "Number of Matches Requested"=1, "error in (no error)"=w404, "Match Color Pattern Setup Data"=w387, "Template Image"=w385, "Image"=w401) -> ("error out"=w402:errorcluster, "Matches"=w390:T8)  [unwired: 3 in, 1 out]
                  n182 = call "overlay_pattern_subVI.vi"("Color"=u32 16774930, "error in"=w402, "Matches"=w390, "Image"=w401) -> ("error out"=w400:errorcluster, "Image Out"=w388:T1)  [unwired: 6 in]
                  n183 = call "IMAQ Match Color Pattern"("Minimum Match Score"="Lip Min Score", "Number of Matches Requested"=1, "error in (no error)"=w400, "Match Color Pattern Setup Data"=w387, "Template Image"=w384, "Image"=w388) -> ("error out"=w399:errorcluster, "Matches"=w389:T8)  [unwired: 3 in, 1 out]
                  n184 = First Call?() -> (First Call?: T/F=w366:bool)
                  n185 = call "face_check_subVI.vi"("Lips Match"=w389, "Nose Match"=w390, "Eye Match"=w391) -> ("Lip Position"=w383:cluster{"x":sgl, "y":sgl}, "Face Found"=w353:bool)  [unwired: 6 in, 1 out]
                  "Face Recognized?" <- w353
                  n186 = Or(x=w366, y=w353) -> (x .or. y?=w367:bool)
                  n187 = call "overlay_pattern_subVI.vi"("Color"=u32 65289, "error in"=w399, "Matches"=w389, "Image"=w388) -> ("error out"=w376:errorcluster, "Image Out"=w378:T1)  [unwired: 6 in]
                  n188 = case shown="False" w367 {
                    tunnel: w415 -> [w428 _]
                    tunnel: w413 -> [w427 _]
                    tunnel: [w426 w429] -> w380
                    tunnel: w411 -> [w425 w432]
                    tunnel: w410 -> [w422 w431]
                    tunnel: [w424 w431] -> w409
                    tunnel: [w423 w432] -> w372
                    tunnel: w383 -> [_ w430]
                    frame False {
                      # "12."
                      n189 = call "IMAQ Optical Flow (LKP)"("error in (no error)"=w425, "Feature Points In"=w427, "Previous Frame"=w428, "Current Frame"=w422) -> ("error out"=w423:errorcluster, "Feature Points Out"=w426:cluster{"X":sgl, "Y":sgl}[], "Current Frame Out (dup)"=w424:T1)  [unwired: 2 in, 3 out]
                    }
                    frame True {
                      n190 = Build Array(w430) -> (w429:cluster{"x":sgl, "y":sgl}[])
                    }
                  }
                  n191 = case shown="False" "Show Templates" {
                    tunnel: w378 -> [w419 w421]
                    tunnel: [w418 w421] -> w377
                    tunnel: w376 -> [w417 w420]
                    tunnel: [w416 w420] -> w374
                    frame False {
                      n192 = call "IMAQ Clear Overlay"("error in (no error)"=w417, "Image"=w419) -> ("error out"=w416:errorcluster, "Image Out"=w418:T1)  [unwired: 8 in]
                    }
                    frame True {
                    }
                  }
                  n193 = call "draw_feature_subVI.vi"("Color"=u32 16711422, "Error In"=w374, "Feature Ponts"=w380, "Image"=w377) -> ("Error Out"=w368:errorcluster, "Image Out"=→"Preview":T1)  [unwired: 6 out]
                  n194 = call "IMAQ Copy"("error in (no error)"=w372, "Image Dst"=w415, "Image Src"=w409) -> ("error out"=w369:errorcluster, "Image Dst Out"=w414:T1)  [unwired: 3 out]
                  n195 = call "Display Message to User"("Enable"=w353) -> ()  [unwired: 9 in, 2 out]
                  n196 = Compound Arithmetic op=OR(w369, w353, w368) -> (w370:bool)
                }
                n197 = Merge Errors(w328, w327) -> (w326:errorcluster)
                n198 = call-poly <vilib>:"Kinect Close.vi"("Kinect References in"=w351, "error in"=w326) -> ("error out"=w334:errorcluster)  [unwired: 13 in]
                n199 = call "IMAQ Dispose"("All Images? (No)"=TRUE, "error in (no error)"=w334) -> ("error out"=w333:errorcluster)  [unwired: 1 in, 3 out]
                n200 = call <vilib>:"Simple Error Handler.vi"("error in (no error)"=w333) -> ()  [unwired: 1 in, 8 out]
              }
            }
          }
          frame "box" {
            n201 = flat-sequence {
              frame #0 {
                w439 = 1 items=["Undefined", "RgbResolution640x480Fps30", "RgbResolution1280x960Fps12", "YuvResolution640x480Fps15", "RawYuvResolution640x480Fps15"]  # RGB Stream Format
                w438 = TRUE  # Skeleton Smoothing
                n202 = call <vilib>:"Initialise.vi"() -> ("Kinect References out"=w434:T3, "error out"=w435:errorcluster)  [unwired: 14 in]
                n203 = call-poly <vilib>:"Configure.vi"("Kinect References in"=w434, "RGB Stream Format"=w439, "Skeleton Smoothing"=w438, "error in"=w435) -> ("Kinect References out"=w440:T4, "error out"=w441:errorcluster)  [unwired: 10 in]
                n204 = call <vilib>:"Initialise 3D Skeleton.vi"("error in (no error)"=w441) -> ("error out"=w442:errorcluster, "Scene & Skeleton Refs"=w443:T5)  [unwired: 9 in]
                n205 = for {
                  N: 300 -> [_]
                  tunnel: [w604] -> w436
                  tunnel: w443 -> [w611]
                  tunnel: w440 -> [w605]
                  shift-right: [w563] -> w437
                  shift-left: w442 -> [w607]
                  w609 = u32 60  # dT
                  n206 = Wait Until Next ms Multiple(millisecond multiple=w609) -> ()  [unwired: 1 out]
                  n207 = call-poly <vilib>:"Read.vi"("Kinect References in"=w605, "error in (no error)"=w607) -> ("Primary Skeleton Array"=w603:dbl[][], "Colour output array (U24, RGB)"=w602:u32[][], "Kinect References out"=w604:T4, "error out"=w606:errorcluster)  [unwired: 9 in, 1 out]
                  n208 = call <vilib>:"Display Colour Data (U32 to picture).vi"("Colour output array (U24, RGB)"=w602) -> ("new picture"=→"measure 2D":picture)  [unwired: 10 in]
                  n209 = call <vilib>:"Render 3D Skeleton.vi"("error in (no error)"=w606, "Array of Joint Positions"=w603, "Scene & Skeleton Refs In"=w611) -> ("error out"=w563:errorcluster, "Array of Joint Positions Out"=w562:dbl[][], "Scene Out"=→"measure 3D":refnum<vi>)  [unwired: 5 in, 1 out]
                  n210 = call <vilib>:"Displacement and Distance Between Joints.vi"("Array of Joint Positions"=w562, "Joint 1"=T2."shoulder centre", "Joint 2"=T2."shoulder left", "error in (no error)"=w563) -> ("X Y Z Displacement Between Joints 1 and 2"=w553:dbl[])  [unwired: 10 in, 1 out]
                  n211 = call <vilib>:"Displacement and Distance Between Joints.vi"("Array of Joint Positions"=w562, "Joint 1"=T2."shoulder left", "Joint 2"=T2."elbow left", "error in (no error)"=w563) -> ("X Y Z Displacement Between Joints 1 and 2"=w550:dbl[])  [unwired: 10 in, 1 out]
                  n212 = call <vilib>:"Displacement and Distance Between Joints.vi"("Array of Joint Positions"=w562, "Joint 1"=T2."elbow left", "Joint 2"=T2."wrist left", "error in (no error)"=w563) -> ("X Y Z Displacement Between Joints 1 and 2"=w544:dbl[])  [unwired: 10 in, 1 out]
                  n213 = call <vilib>:"Displacement and Distance Between Joints.vi"("Array of Joint Positions"=w562, "Joint 1"=T2."ankle left", "Joint 2"=T2."foot left", "error in (no error)"=w563) -> ("X Y Z Displacement Between Joints 1 and 2"=w517:dbl[])  [unwired: 10 in, 1 out]
                  n214 = call <vilib>:"Displacement and Distance Between Joints.vi"("Array of Joint Positions"=w562, "Joint 1"=T2."knee left", "Joint 2"=T2."ankle left", "error in (no error)"=w563) -> ("X Y Z Displacement Between Joints 1 and 2"=w518:dbl[])  [unwired: 10 in, 1 out]
                  n215 = call <vilib>:"Displacement and Distance Between Joints.vi"("Array of Joint Positions"=w562, "Joint 1"=T2."wrist left", "Joint 2"=T2."hand left", "error in (no error)"=w563) -> ("X Y Z Displacement Between Joints 1 and 2"=w534:dbl[])  [unwired: 10 in, 1 out]
                  n216 = call <vilib>:"Displacement and Distance Between Joints.vi"("Array of Joint Positions"=w562, "Joint 1"=T2."hip left", "Joint 2"=T2."knee left", "error in (no error)"=w563) -> ("X Y Z Displacement Between Joints 1 and 2"=w519:dbl[])  [unwired: 10 in, 1 out]
                  n217 = call <vilib>:"Displacement and Distance Between Joints.vi"("Array of Joint Positions"=w562, "Joint 1"=T2."hip centre", "Joint 2"=T2."hip left", "error in (no error)"=w563) -> ("X Y Z Displacement Between Joints 1 and 2"=w526:dbl[])  [unwired: 10 in, 1 out]
                  n218 = Square(x=w534) -> (x^2=w538:dbl[])
                  n219 = Square(x=w553) -> (x^2=w555:dbl[])
                  n220 = Square(x=w550) -> (x^2=w552:dbl[])
                  n221 = Square(x=w518) -> (x^2=w523:dbl[])
                  n222 = Square(x=w517) -> (x^2=w521:dbl[])
                  n223 = Square(x=w544) -> (x^2=w546:dbl[])
                  n224 = Square(x=w519) -> (x^2=w525:dbl[])
                  n225 = Square(x=w526) -> (x^2=w528:dbl[])
                  n226 = Add Array Elements(numeric array=w538) -> (sum=w537:dbl)
                  n227 = Add Array Elements(numeric array=w555) -> (sum=w554:dbl)
                  n228 = Add Array Elements(numeric array=w552) -> (sum=w551:dbl)
                  n229 = Add Array Elements(numeric array=w523) -> (sum=w522:dbl)
                  n230 = Add Array Elements(numeric array=w521) -> (sum=w520:dbl)
                  n231 = Add Array Elements(numeric array=w546) -> (sum=w545:dbl)
                  n232 = Add Array Elements(numeric array=w525) -> (sum=w524:dbl)
                  n233 = Add Array Elements(numeric array=w528) -> (sum=w527:dbl)
                  n234 = Square Root(x=w537) -> (sqrt(x)=w487:dbl)
                  n235 = Square Root(x=w554) -> (sqrt(x)=w495:dbl)
                  n236 = Square Root(x=w551) -> (sqrt(x)=w492:dbl)
                  n237 = Square Root(x=w522) -> (sqrt(x)=w460:dbl)
                  n238 = Square Root(x=w520) -> (sqrt(x)=w457:dbl)
                  n239 = Square Root(x=w545) -> (sqrt(x)=w489:dbl)
                  n240 = Multiply(x=w487, y=100.0) -> (x*y=w486:dbl)
                  n241 = Square Root(x=w524) -> (sqrt(x)=w463:dbl)
                  n242 = Square Root(x=w527) -> (sqrt(x)=w466:dbl)
                  n243 = Multiply(x=w495, y=100.0) -> (x*y=w496:dbl)
                  n244 = Multiply(x=w489, y=100.0) -> (x*y=w490:dbl)
                  n245 = Multiply(x=w492, y=100.0) -> (x*y=w493:dbl)
                  n246 = Multiply(x=w460, y=100.0) -> (x*y=w459:dbl)
                  n247 = Multiply(x=w463, y=100.0) -> (x*y=w462:dbl)
                  n248 = Multiply(x=w457, y=100.0) -> (x*y=w456:dbl)
                  n249 = Multiply(x=w466, y=100.0) -> (x*y=w465:dbl)
                  n250 = call <vilib>:"Displacement and Distance Between Joints.vi"("Array of Joint Positions"=w562, "Joint 1"=T2."head", "Joint 2"=T2."shoulder centre", "error in (no error)"=w563) -> ("X Y Z Displacement Between Joints 1 and 2"=w559:dbl[])  [unwired: 10 in, 1 out]
                  n251 = Square(x=w559) -> (x^2=w561:dbl[])
                  n252 = Add Array Elements(numeric array=w561) -> (sum=w560:dbl)
                  n253 = Square Root(x=w560) -> (sqrt(x)=w498:dbl)
                  n254 = call <vilib>:"Displacement and Distance Between Joints.vi"("Array of Joint Positions"=w562, "Joint 1"=T2."shoulder centre", "Joint 2"=T2."spine", "error in (no error)"=w563) -> ("X Y Z Displacement Between Joints 1 and 2"=w532:dbl[])  [unwired: 10 in, 1 out]
                  n255 = call <vilib>:"Displacement and Distance Between Joints.vi"("Array of Joint Positions"=w562, "Joint 1"=T2."spine", "Joint 2"=T2."hip centre", "error in (no error)"=w563) -> ("X Y Z Displacement Between Joints 1 and 2"=w529:dbl[])  [unwired: 10 in, 1 out]
                  n256 = Square(x=w532) -> (x^2=w540:dbl[])
                  n257 = Square(x=w529) -> (x^2=w531:dbl[])
                  n258 = Add Array Elements(numeric array=w540) -> (sum=w539:dbl)
                  n259 = Add Array Elements(numeric array=w531) -> (sum=w530:dbl)
                  n260 = Square Root(x=w539) -> (sqrt(x)=w484:dbl)
                  n261 = Multiply(x=w498, y=100.0) -> (x*y=w499:dbl)
                  n262 = Square Root(x=w530) -> (sqrt(x)=w480:dbl)
                  n263 = Multiply(x=w484, y=100.0) -> (x*y=w483:dbl)
                  n264 = Multiply(x=w480, y=100.0) -> (x*y=w481:dbl)
                  n265 = call <vilib>:"Displacement and Distance Between Joints.vi"("Array of Joint Positions"=w562, "Joint 1"=T2."shoulder centre", "Joint 2"=T2."shoulder right", "error in (no error)"=w563) -> ("X Y Z Displacement Between Joints 1 and 2"=w556:dbl[])  [unwired: 10 in, 1 out]
                  n266 = call <vilib>:"Displacement and Distance Between Joints.vi"("Array of Joint Positions"=w562, "Joint 1"=T2."shoulder right", "Joint 2"=T2."elbow right", "error in (no error)"=w563) -> ("X Y Z Displacement Between Joints 1 and 2"=w547:dbl[])  [unwired: 10 in, 1 out]
                  n267 = call <vilib>:"Displacement and Distance Between Joints.vi"("Array of Joint Positions"=w562, "Joint 1"=T2."elbow right", "Joint 2"=T2."wrist right", "error in (no error)"=w563) -> ("X Y Z Displacement Between Joints 1 and 2"=w541:dbl[])  [unwired: 10 in, 1 out]
                  n268 = Square(x=w556) -> (x^2=w558:dbl[])
                  n269 = call <vilib>:"Displacement and Distance Between Joints.vi"("Array of Joint Positions"=w562, "Joint 1"=T2."wrist right", "Joint 2"=T2."hand right", "error in (no error)"=w563) -> ("X Y Z Displacement Between Joints 1 and 2"=w533:dbl[])  [unwired: 10 in, 1 out]
                  n270 = Square(x=w547) -> (x^2=w549:dbl[])
                  n271 = Add Array Elements(numeric array=w558) -> (sum=w557:dbl)
                  n272 = call <vilib>:"Displacement and Distance Between Joints.vi"("Array of Joint Positions"=w562, "Joint 1"=T2."hip centre", "Joint 2"=T2."hip right", "error in (no error)"=w563) -> ("X Y Z Displacement Between Joints 1 and 2"=w514:dbl[])  [unwired: 10 in, 1 out]
                  n273 = Square(x=w541) -> (x^2=w543:dbl[])
                  n274 = call <vilib>:"Displacement and Distance Between Joints.vi"("Array of Joint Positions"=w562, "Joint 1"=T2."hip right", "Joint 2"=T2."knee right", "error in (no error)"=w563) -> ("X Y Z Displacement Between Joints 1 and 2"=w507:dbl[])  [unwired: 10 in, 1 out]
                  n275 = call <vilib>:"Displacement and Distance Between Joints.vi"("Array of Joint Positions"=w562, "Joint 1"=T2."knee right", "Joint 2"=T2."ankle right", "error in (no error)"=w563) -> ("X Y Z Displacement Between Joints 1 and 2"=w506:dbl[])  [unwired: 10 in, 1 out]
                  n276 = call <vilib>:"Displacement and Distance Between Joints.vi"("Array of Joint Positions"=w562, "Joint 1"=T2."ankle right", "Joint 2"=T2."foot right", "error in (no error)"=w563) -> ("X Y Z Displacement Between Joints 1 and 2"=w505:dbl[])  [unwired: 10 in, 1 out]
                  n277 = Square(x=w533) -> (x^2=w536:dbl[])
                  n278 = Add Array Elements(numeric array=w549) -> (sum=w548:dbl)
                  n279 = Square Root(x=w557) -> (sqrt(x)=w478:dbl)
                  n280 = Add Array Elements(numeric array=w543) -> (sum=w542:dbl)
                  n281 = Add Array Elements(numeric array=w536) -> (sum=w535:dbl)
                  n282 = Square Root(x=w548) -> (sqrt(x)=w474:dbl)
                  n283 = Square Root(x=w542) -> (sqrt(x)=w472:dbl)
                  n284 = Square(x=w506) -> (x^2=w511:dbl[])
                  n285 = Square(x=w507) -> (x^2=w513:dbl[])
                  n286 = Square(x=w505) -> (x^2=w508:dbl[])
                  n287 = Square(x=w514) -> (x^2=w516:dbl[])
                  n288 = Square Root(x=w535) -> (sqrt(x)=w469:dbl)
                  n289 = Add Array Elements(numeric array=w511) -> (sum=w510:dbl)
                  n290 = Add Array Elements(numeric array=w513) -> (sum=w512:dbl)
                  n291 = Add Array Elements(numeric array=w508) -> (sum=w509:dbl)
                  n292 = Add Array Elements(numeric array=w516) -> (sum=w515:dbl)
                  n293 = Multiply(x=w478, y=100.0) -> (x*y=w477:dbl)
                  n294 = Square Root(x=w510) -> (sqrt(x)=w450:dbl)
                  n295 = Multiply(x=w474, y=100.0) -> (x*y=w475:dbl)
                  n296 = Square Root(x=w512) -> (sqrt(x)=w448:dbl)
                  n297 = Square Root(x=w509) -> (sqrt(x)=w453:dbl)
                  n298 = Square Root(x=w515) -> (sqrt(x)=w445:dbl)
                  n299 = Multiply(x=w472, y=100.0) -> (x*y=w471:dbl)
                  n300 = Multiply(x=w469, y=100.0) -> (x*y=w468:dbl)
                  n301 = Multiply(x=w445, y=100.0) -> (x*y=w444:dbl)
                  n302 = Multiply(x=w453, y=100.0) -> (x*y=w454:dbl)
                  n303 = Multiply(x=w450, y=100.0) -> (x*y=w451:dbl)
                  n304 = Multiply(x=w448, y=100.0) -> (x*y=w447:dbl)
                  n305 = Build Array(w481, w483, w499, w496, w493, w490, w486, w477, w475, w471, w468, w465, w462, w459, w456, w444, w447, w451, w454) -> (w501:dbl[])
                  "real time data" <- w501
                  n306 = Array Size(array=w501) -> ()  [unwired: 1 out]
                  n307 = call-poly <vilib>:"Write Delimited Spreadsheet.vi"("file path (dialog if empty)"=path "D:/skeleton data.csv", "1D data"=w501, "append to file? (new file:F)"=TRUE, "delimiter (\\t)"="," ("delimiter (\\t)")) -> ()  [unwired: 10 in, 2 out]
                }
                n308 = call-poly <vilib>:"Kinect Close.vi"("Kinect References in"=w436, "error in"=w437) -> ()  [unwired: 13 in, 1 out]
              }
              frame #1 {
                n309 = call-poly <vilib>:"Read Delimited Spreadsheet.vi"("file path (dialog if empty)"=path "D:/skeleton data.csv" ("file path (dialog if empty) 2"), "format (%.3f)"="%d", "transpose? (F)"=FALSE, "delimiter (\\t)"="," ("delimiter (\\t)")) -> ("all rows"=w623:dbl[][])  [unwired: 6 in, 5 out]
                n310 = Array Size(array=w623) -> ()  [unwired: 1 out]
                n311 = for "takes the columns 1 by one and checks if it's full of zeros" {
                  tunnel: w623 -> [w635] mode=indexing
                  shift-right: [w633] -> w624
                  shift-left: _ -> [w634]
                  i -> [w632]
                  n312 = Equal To 0?(x=w635) -> (x = 0?=w631:bool[])
                  n313 = And Array Elements(Boolean array=w631) -> (logical AND=w630:bool)
                  n314 = case "keep the index of \"off-devices\"" shown="True" w630 {
                    tunnel: w634 -> [w636 w637]
                    tunnel: [w636 w639] -> w633
                    tunnel: w632 -> [_ w638]
                    frame False {
                    }
                    frame True {
                      n315 = Build Array (concatenate)(w638, w637) -> (w639:i32[])
                    }
                  }
                }
                n316 = for "remove column you don't want" {
                  shift-right: [w628] -> w619
                  shift-left: w623 -> [w629]
                  tunnel: w624 -> [w627] mode=indexing
                  n317 = Delete From Array(array=w629, index (row)=w627) -> (array with subset deleted=w628:dbl[][])  [unwired: 2 in, 1 out]
                }
                n318 = Array Size(array=w619) -> (size(s)=w621:i32[])
                n319 = Index Array(array=w621, index=1) -> (element=w620:i32)
                n320 = for {
                  N: w620 -> [_]
                  tunnel: w619 -> [w643]
                  tunnel: [w640] -> w617 mode=indexing
                  i -> [w642]
                  n321 = Index Array(array=w643, index (col)=w642) -> (element=w641:dbl[])  [unwired: 1 in]
                  n322 = call-poly <vilib>:"Mean.vi"("X"=w641) -> ("mean"=w640:dbl)  [unwired: 1 out]
                }
                "mean calculated" <- w617
                n323 = call-poly <vilib>:"Write Delimited Spreadsheet.vi"("file path (dialog if empty)"=path "D:/mean.csv" ("file path (dialog if empty) 3"), "format (%.3f)"="%.3f", "1D data"=w617, "transpose? (no:F)"=TRUE, "delimiter (\\t)"="," ("delimiter (\\t)")) -> ()  [unwired: 9 in, 2 out]
              }
            }
          }
        }
      }
    }
  }
  "Error Out" <- w3
